vi "System Beep.vi"(1 "icon (0:None)":i32(ring)) -> ()   [LabVIEW 2011]
uses:
  user32.dll
panel:
  in  "icons":i32[](array[numeric])=[0, 16, 32, 48, 64, 5, 16, 32, 48, 64] format="%.0x"
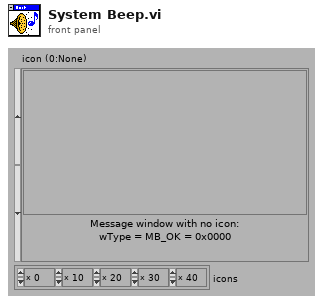
[diagram p1: front panel]
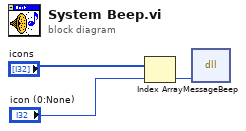
[diagram p0: block diagram]
diagram:
  n1 = Index Array(array="icons", index="icon (0:None)") -> (element=w1:i32)
  n2 = dll-call lib="User32.dll" fn="MessageBeep"("wType"=w1) -> ()  [unwired: 4 in, 3 out]
